vi "List All Ctrls.vi"(8 "error in (no error)":errorcluster, 11 "VI Refnum":refnum<vi>) -> (0 "error out":errorcluster, 1 "Indicators":refnum<vi>[](array[refnum]), 2 "Ctrls":refnum<vi>[](array[refnum]), 3 "VI Refnum (dup)":refnum<vi>)   [LabVIEW 2017]
panel:
  out "?":refnum<vi>
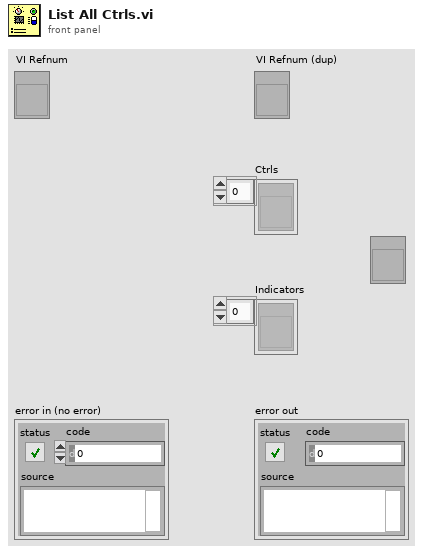
[diagram p1: front panel]
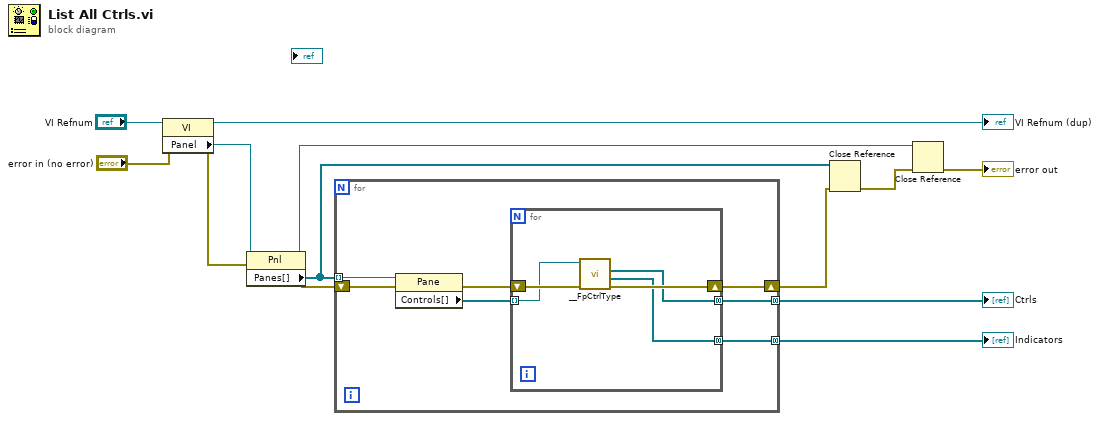
[diagram p0: block diagram]
diagram:
  n1 = property on="Property Node" class="VI"(reference="VI Refnum", error in="error in (no error)") -> (reference out=→"VI Refnum (dup)":refnum<vi>, error out=w10:errorcluster, "Panel"=w11:refnum<vi>)
  n2 = property on="Property Node" class="Pnl"(reference=w11, error in=w10) -> (reference out=w8:refnum<vi>, error out=w9:errorcluster, "Panes[]"=w7:refnum<vi>[])
  n3 = for {
    tunnel: w7 -> [w20] mode=indexing
    tunnel: [w18] -> w2 mode=concatenating
    tunnel: [w17] -> w1 mode=concatenating
    shift-right: [w14] -> w6
    shift-left: w9 -> [w16]
    n4 = property class="Pane"(reference=w20, error in=w16) -> (error out=w15:errorcluster, "Controls[]"=w19:refnum<vi>[])  [unwired: 1 out]
    n5 = for {
      tunnel: w19 -> [w23] mode=indexing
      tunnel: [w22] -> w18 mode=concatenating
      tunnel: [w21] -> w17 mode=concatenating
      shift-right: [w25] -> w14
      shift-left: w15 -> [w24]
      n6 = call "__FpCtrlType.vi"("error out"=w24, "reference"=w23) -> ("error out 2"=w25:errorcluster, "ControlsIndicator"=w21:refnum<vi>[], "Controls"=w22:refnum<vi>[])  [unwired: 6 in, 1 out]
    }
  }
  "Ctrls" <- w2
  "Indicators" <- w1
  n7 = Close Reference(reference=w7, error in (no error)=w6) -> (error out=w5:errorcluster)
  n8 = Close Reference(reference=w8, error in (no error)=w5) -> (error out=→"error out":errorcluster)
